vi "Read ProtocolConfig.vi"(8 "error in (no error)":errorcluster, 11 "Protocol in":refnum<class "Protocol.lvclass">) -> (0 "error out":errorcluster, 2 "ProtocolConfig.lvclass":refnum<class "ProtocolConfig.lvclass">, 3 "Protocol out":refnum<class "Protocol.lvclass">)   [LabVIEW 2020, in "FileSync -- Base.lvlib" / "Protocol.lvclass"]
uses:
  Protocol.lvclass
  ProtocolConfig/ProtocolConfig.lvclass
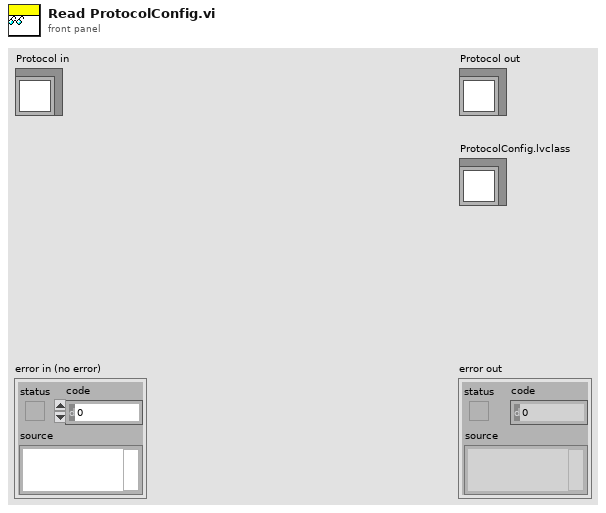
[diagram p1: front panel]
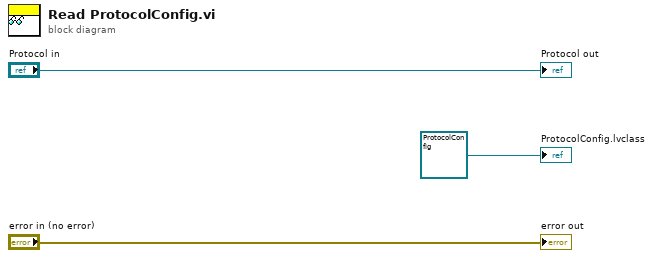
[diagram p0: block diagram]
diagram:
  "error out" <- "error in (no error)"
  "Protocol out" <- "Protocol in"
  "ProtocolConfig.lvclass" <- refnum<class "ProtocolConfig.lvclass"> refnum ("ProtocolConfig.lvclass")
